vi "terminate.vi"(8 "error in (no error)":errorcluster, 11 "GenericPlugin in":refnum<class "StageFH090410SharedVariable.lvclass">) -> (0 "error out":errorcluster, 3 "GenericPlugin out":refnum<class "StageFH090410SharedVariable.lvclass">)   [LabVIEW 2010, in "StageFH090410SharedVariable.lvclass"]
doc: "The dynamic dispatch version of this VI terminates the plug-in object by releasing all of its resources."
uses:
  StageFH090410SharedVariable.lvclass
  StageFH090410SharedVariable.lvclass/StageFH090410SharedVariable.ctl
  StageDL090409Scaffold/StageDL090409Scaffold/StageDL090409Scaffold.lvclass
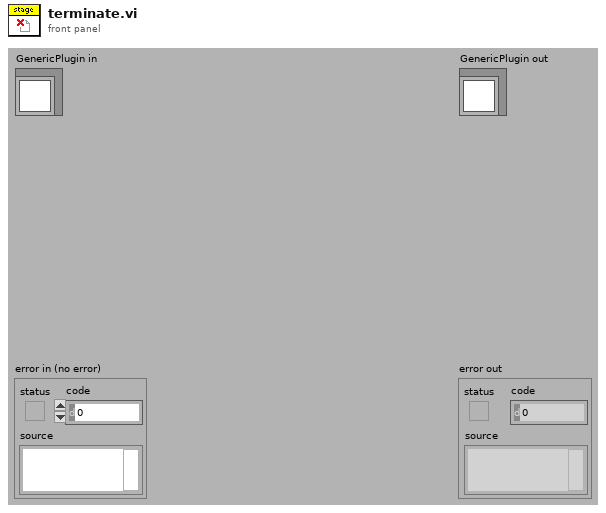
[diagram p1: front panel]
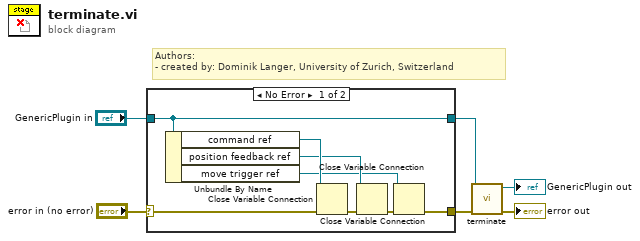
[diagram p0: block diagram]
diagram:
  # "Authors: \n- created by: Dominik Langer, University of Zurich, Switzerland"
  n1 = case shown="No Error" "error in (no error)" {
    selector: "error in (no error)" -> [w14 w16]
    tunnel: [w8 w16] -> w3
    tunnel: [w7 w15] -> w1
    tunnel: "GenericPlugin in" -> [w7 w15]
    frame No Error {
      n2 = Unbundle By Name(w7) -> ("command ref"=w13:refnum<k21>, "position feedback ref"=w12:refnum<k21>, "move trigger ref"=w11:refnum<k21>)
      n3 = Close Variable Connection(8:w14, 11:w13) -> (0:w10:errorcluster)
      n4 = Close Variable Connection(8:w10, 11:w12) -> (0:w9:errorcluster)
      n5 = Close Variable Connection(8:w9, 11:w11) -> (0:w8:errorcluster)
    }
    frame Error {
    }
  }
  n6 = call-parent "terminate.vi"("error in (no error)"=w3, "GenericPlugin in"=w1) -> ("error out"=→"error out":errorcluster, "GenericPlugin out"=→"GenericPlugin out":refnum<class "StageFH090410SharedVariable.lvclass">)  [unwired: 8 in]
